vi "GV status converter.vi"(11 "Gate Valve":T1) -> (3 "GV Status":T2)   [LabVIEW 2016]
doc: "Converts position sensor data to a state:\nGV open (OPEN sensor = TRUE; closed sensor = FALSE)\nGV out (OPEN sensor = FALSE; closed sensor = TRUE)\nGV status unclear (OPEN sensor = closed sensor)"
uses:
  Controls/GV states.ctl
  Controls/Gate Valve Readback.ctl
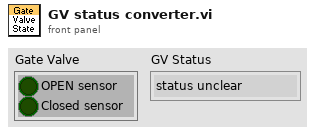
[diagram p1: front panel]
types:
  T1 = typedef "Gate Valve Readback.ctl" = cluster{"OPEN sensor":bool, "Closed sensor":bool}
  T2 = typedef "GV states.ctl" = enum16{"status unclear", "closed", "open"}
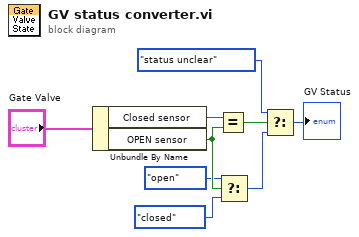
[diagram p0: block diagram]
diagram:
  n1 = Unbundle By Name("Gate Valve") -> ("Closed sensor"=w6:bool, "OPEN sensor"=w8:bool)
  n2 = Equal?(x=w6, y=w8) -> (x = y?=w7:bool)
  n3 = Select(t=GV_states."open" ("Enum"), s=w8, f=GV_states."closed" ("Enum")) -> (s? t:f=w9:T2)
  n4 = Select(t=GV_states."status unclear" ("Enum"), s=w7, f=w9) -> (s? t:f=→"GV Status":T2)
